vi "PROTECAO_DEC.vi"() -> (3 "CONT DEC":i32)   [LabVIEW 2018]
uses:
  Global_Telescopio.vi
panel:
  out "DIST DEC":dbl
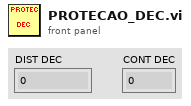
[diagram p1: front panel]
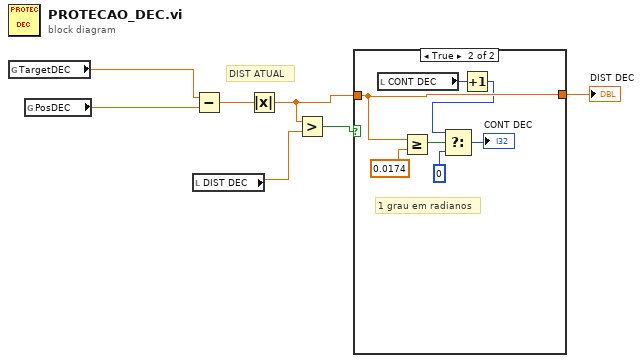
[diagram p0: block diagram]
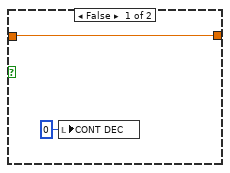
[diagram p2: hidden frame]
diagram:
  # "DIST ATUAL"
  n1 = global read "Global_Telescopio.vi" "TargetDEC"() -> (w7:dbl)
  n2 = global read "Global_Telescopio.vi" "PosDEC"() -> (w6:dbl)
  n3 = local read "DIST DEC"() -> (w2:dbl)
  n4 = Subtract(x=w7, y=w6) -> (x-y=w5:dbl)
  n5 = Absolute Value(x=w5) -> (abs(x)=w1:dbl)
  n6 = Greater?(x=w1, y=w2) -> (0:w3:bool)
  n7 = case shown="True" w3 {
    tunnel: w1 -> [w9 w16]
    tunnel: [w9 w16] -> w4
    frame False {
      n8 = local write "CONT DEC"(0 ("CONT AH")) -> ()
    }
    frame True {
      # "1 grau em radianos"
      n9 = local read "CONT DEC"() -> (w11:i32)
      n10 = Greater Or Equal?(x=w16, y=0.0174) -> (x >= y?=w14:bool)
      n11 = Increment(x=w11) -> (x+1=w10:i32)
      n12 = Select(t=w10, s=w14, f=0 ("t")) -> (s? t:f=→"CONT DEC":i32)
    }
  }
  "DIST DEC" <- w4
